vi "7. FGV Data check.vi"(8 "error in (no error)":errorcluster, 9 "cmd type (CMD = 0, ACK = 1, NAK = 2)":u32, 10 "Cnt":u32, 11 "VISA resource name":refnum<visa-resource-name>="COM3") -> (0 "error out":errorcluster, 1 "Checksum":u32, 2 "Error":i32, 3 "Data":i32[](array[numeric]))   [LabVIEW 2014]
uses:
  control/FGV Serial Tasks.ctl
panel:
  out "return count":u32
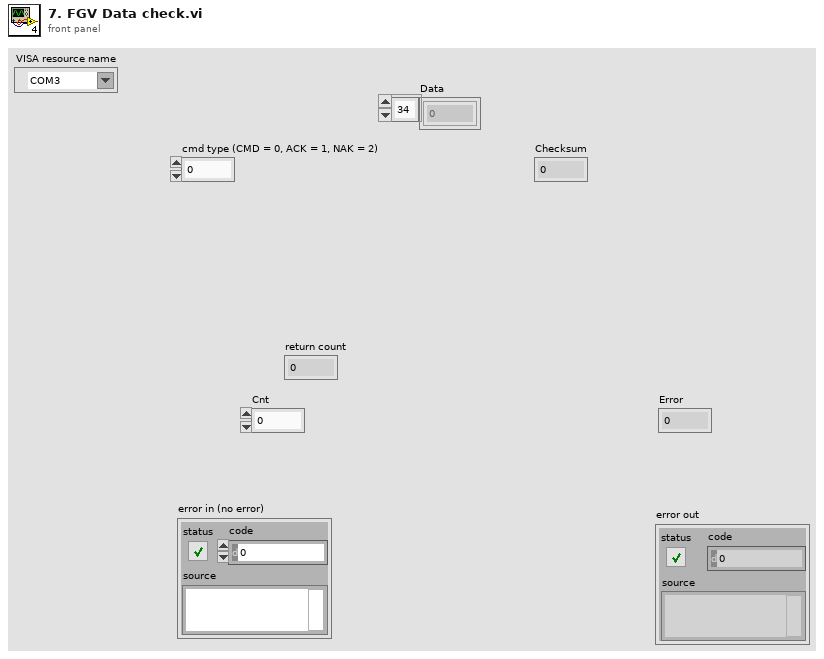
[diagram p1: front panel]
types:
  T1 = typedef "FGV Serial Tasks.ctl" = enum16{"Open", "Read", "Write", "Close", "Flush"}
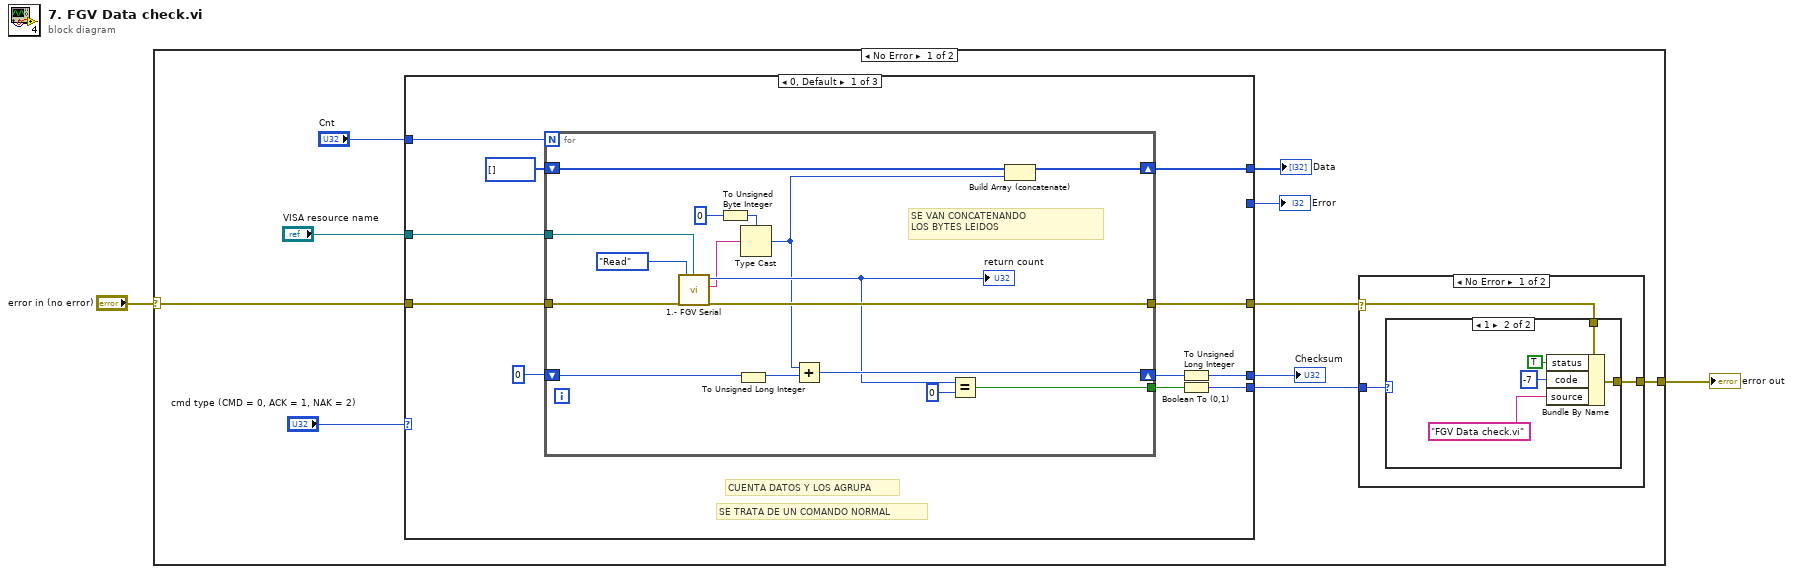
[diagram p0: block diagram]
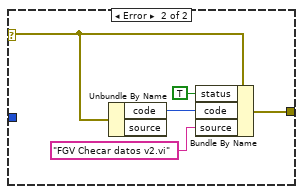
[diagram p3: hidden frame]
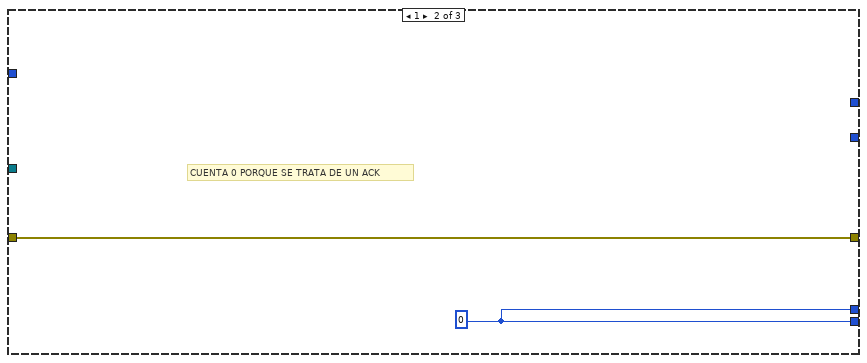
[diagram p4: hidden frame]
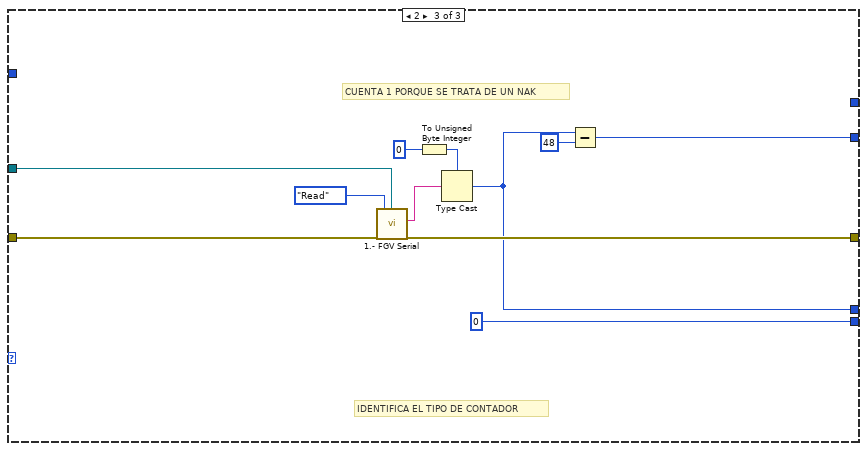
[diagram p5: hidden frame]
diagram:
  n1 = case shown="No Error" "error in (no error)" {
    selector: "error in (no error)" -> [w12 w67]
    tunnel: [w9 w67] -> w1
    frame No Error {
      n2 = case shown="0, Default" "cmd type (CMD = 0, ACK = 1, NAK = 2)" {
        tunnel: w12 -> [w37 w54 w66]
        tunnel: [w36 w54 w65] -> w10
        tunnel: [w35 w55 w63] -> w11
        tunnel: [w34 w55 i16 0] -> w8
        tunnel: "VISA resource name" -> [w33 _ w62]
        tunnel: "Cnt" -> [w28 _ _]
        tunnel: [w27 _ _] -> w4
        tunnel: [_ _ w56] -> w3
        frame 0, Default {
          # "CUENTA DATOS Y LOS AGRUPA"
          # "SE TRATA DE UN COMANDO NORMAL"
          n3 = for {
            N: w28 -> [_]
            tunnel: w37 -> [w53]
            tunnel: [w52] -> w36
            shift-right: [w51] -> w31
            shift-left: u32 0 ("y") -> [w46]
            tunnel: [w48] -> w30
            shift-right: [w45] -> w27
            shift-left: i32[] [] -> [w44]
            tunnel: w33 -> [w42]
            # "SE VAN CONCATENANDO\nLOS BYTES LEIDOS"
            n4 = call "1.- FGV Serial.vi"("VISA resource name"=w42, "error in (no error)"=w53, "Task"=FGV_Serial_Tasks."Read") -> ("error out"=w52:errorcluster, "Receive buffer"=w40:string, "return count"=w50:u32)  [unwired: 6 in]
            "return count" <- w50
            n5 = To Unsigned Byte Integer(number=u8 0) -> (unsigned 8bit integer=w39:u8)
            n6 = To Unsigned Long Integer(number=w46) -> (unsigned 32bit integer=w47:u32)
            n7 = Type Cast(type=w39, x=w40) -> (*(type *) &x=w43:u8)
            n8 = Add(x=w43, y=w47) -> (x+y=w51:u32)
            n9 = Equal?(x=w50, y=u32 0) -> (x = y?=w48:bool)
            n10 = Build Array (concatenate) "Build Array"(w44, w43) -> (w45:i32[])
          }
          n11 = To Unsigned Long Integer(number=w31) -> (unsigned 32bit integer=w35:u32)
          n12 = Boolean To (0,1)(Boolean=w30) -> (0, 1=w34:i16)
        }
        frame 1 {
          w55 = 0 ("Text output")
          # "CUENTA 0 PORQUE SE TRATA DE UN ACK"
        }
        frame 2 {
          # "CUENTA 1 PORQUE SE TRATA DE UN NAK"
          # "IDENTIFICA EL TIPO DE CONTADOR"
          n13 = call "1.- FGV Serial.vi"("VISA resource name"=w62, "error in (no error)"=w66, "Task"=FGV_Serial_Tasks."Read") -> ("error out"=w65:errorcluster, "Receive buffer"=w59:string)  [unwired: 6 in, 1 out]
          n14 = To Unsigned Byte Integer(number=u8 0) -> (unsigned 8bit integer=w58:u8)
          n15 = Type Cast(type=w58, x=w59) -> (*(type *) &x=w63:u8)
          n16 = Subtract(x=w63, y=48) -> (x-y=w56:i32)
        }
      }
      "Checksum" <- w11
      "Data" <- w4
      "Error" <- w3
      n17 = case shown="No Error" w10 {
        selector: w10 -> [w14 w25]
        tunnel: [w15 w24] -> w9
        tunnel: w8 -> [w13 _]
        frame No Error {
          n18 = case shown="1" w13 {
            tunnel: [w16 w19] -> w15
            tunnel: w14 -> [w16 w18]
            frame 0, Default {
            }
            frame 1 {
              n19 = Bundle By Name(cluster=w18, "status"=TRUE, "code"=-7, "source"="FGV Data check.vi") -> (w19:errorcluster)
            }
          }
        }
        frame Error {
          n20 = Unbundle By Name(w25) -> ("code"=w26:i32)  [unwired: 1 out]
          n21 = Bundle By Name(cluster=w25, "status"=TRUE, "code"=w26, "source"="FGV Checar datos v2.vi") -> (w24:errorcluster)
        }
      }
    }
    frame Error {
    }
  }
  "error out" <- w1
